vi "Close to SFTP.vi"(8 "Error In":errorcluster, 11 "SFTP Directory":refnum<class "SFTP Directory.lvclass">) -> (0 "Error Out":errorcluster, 2 "Remote Path":string, 3 "SFTP":refnum<class "SFTP.lvclass">)   [LabVIEW 2021, in "Field_RnD_Services_LIBSSH2_Toolkit.lvlib" / "SFTP Directory.lvclass"]
doc: "Destroys this SFTP Directory object and returns the SFTP object used to create it."
uses:
  SFTP Directory.lvclass
  SFTP/SFTP.lvclass
  SFTP Directory.lvclass/SFTP Directory.ctl
  Field_RnD_Services_LIBSSH2_Toolkit.lvlib
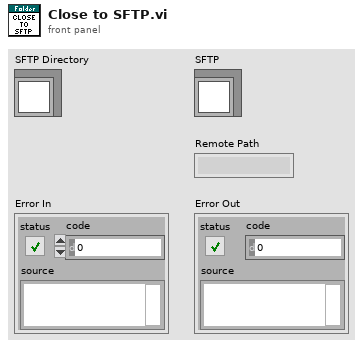
[diagram p1: front panel]
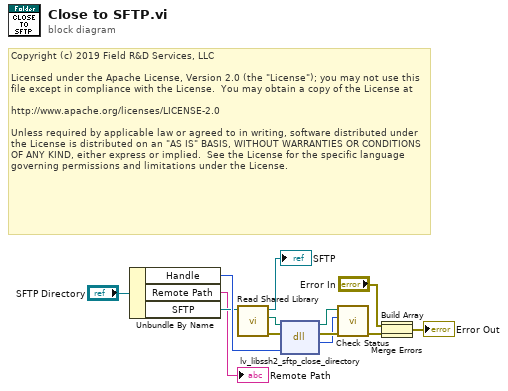
[diagram p0: block diagram]
diagram:
  # "Copyright (c) 2019 Field R&D Services, LLC\n\nLicensed under the Apache License, Version 2.0 (the \"License\"); you may not use this file except in compliance with the License.  You may obtain a copy of the License at\n\nhttp://www.apache.org/licenses/LICENSE-2.0\n\nUnless required by applicable law or agreed to in writing, software distributed under the License is distributed on an \"AS IS\" BASIS, WITHOUT WARRANTIES OR CONDITIONS OF ANY KIND, either express or implied.  See the License for the specific language governing permissions and limitations under the License."
  n1 = Unbundle By Name("SFTP Directory") -> ("Handle"=w12:u64, "Remote Path"=→"Remote Path":string, "SFTP"=w6:refnum<class "SFTP.lvclass">)
  n2 = call "Read Shared Library.vi"("SFTP In"=w6) -> ("Erorr Out"=w3:errorcluster, "libssh2lv Shared Library"=w4:path, "SFTP Out"=→"SFTP":refnum<class "SFTP.lvclass">)  [unwired: 8 in]
  n3 = dll-call lib="lv-libssh2.*" fn="lv_libssh2_sftp_close_directory"(path in=w4, error in=w3, "handle"=w12) -> (path out=w10:path, error out=w11:errorcluster, "status"=w8:i32)  [unwired: 2 in]
  n4 = call "Check Status.vi"("Error In"=w11, "Status"=w8, "libssh2lv Shared Library In"=w10) -> ("Error Out"=w9:errorcluster)  [unwired: 7 in, 1 out]
  n5 = Build Array("Error In", w9) -> (w1:errorcluster[])
  n6 = Merge Errors(w1) -> (→"Error Out":errorcluster)
